vi "config_file_load_create.vi"(0 "configuration file path":path, 1 "reference cluster in":T1, 3 "error in":errorcluster) -> (8 "reference cluster out":T1, 10 "error out":errorcluster)   [LabVIEW 2016]
uses:
  Type Definitions/reference_cluster.ctl
  Type Definitions/vars_settings.ctl
  Type Definitions/stim_type.ctl
  Type Definitions/vars_runtime.ctl
  Type Definitions/data.ctl
  Type Definitions/notifier_elements_GUI.ctl
  Type Definitions/notifier_elements_DAQ.ctl
  Type Definitions/notifier_elements_write.ctl
  Type Definitions/control_references.ctl
  <vilib>/Utility/config.llb/NI_LVConfig.lvlib
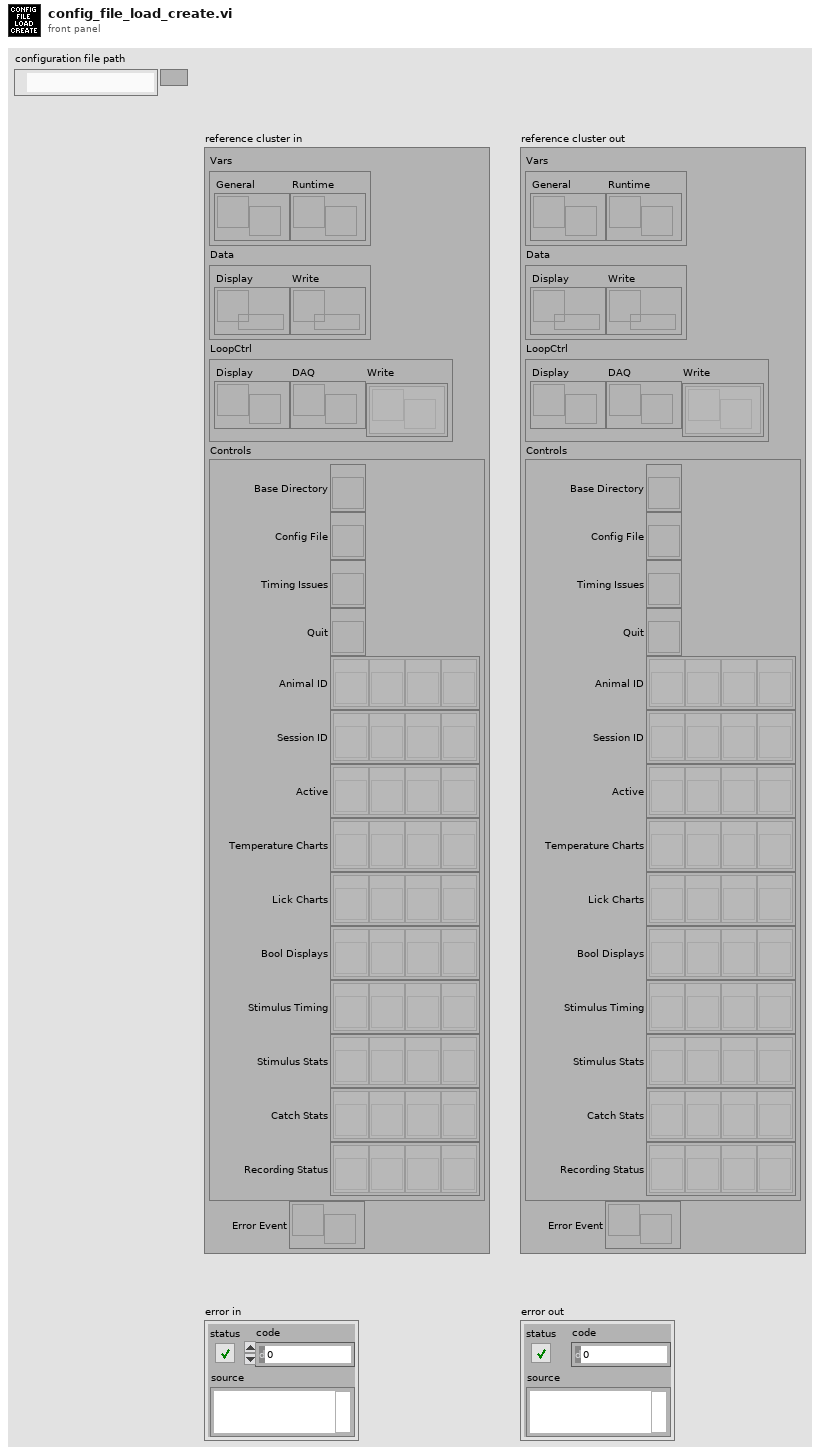
[diagram p1: front panel]
types:
  T1 = typedef "reference_cluster.ctl" = cluster{"Vars":cluster{"General":refnum<notifier>, "Runtime":refnum<notifier>}, "Data":cluster{"Display":refnum<queue>, "Write":refnum<queue>}, "LoopCtrl":cluster{"Display":refnum<notifier>, "DAQ":refnum<notifier>, "Write":refnum<notifier>[]}, "Controls":T2, "Error Event":refnum<user-event>}
  T2 = typedef "control_references.ctl" = cluster{"Base Directory":refnum<vi>, "Config File":refnum<vi>, "Timing Issues":refnum<vi>, "Quit":refnum<vi>, "Animal ID":refnum<vi>[], "Session ID":refnum<vi>[], "Active":refnum<vi>[], "Temperature Charts":refnum<vi>[], "Lick Charts":refnum<vi>[], "Bool Displays":refnum<vi>[], "Stimulus Timing":refnum<vi>[], "Stimulus Stats":refnum<vi>[], "Catch Stats":refnum<vi>[], "Recording Status":refnum<vi>[]}
  T3 = typedef "vars_settings.ctl" = cluster{"base directory":path, "data directory":path, "active":bool, "running":bool, "pairing":bool, "clean tubes":bool, "animal ID":u16, "session ID":u16, "base temp":dbl, "d wait min":u16, "d wait max":u16, "d timeout":u16, "d reward":u16, "idx stim":u16, "timeout win":u16, "lick win":i32[], "stim type":T4[], "stim amps":dbl[], "d stim":u16[], "d ramp":u16[], "f vibration":u16[], "f squarewave":u8[], "stim shape":dbl[][], "catch":u8[]}
  T4 = typedef "stim_type.ctl" = enum16{"pulse", "vibration", "square", "sine"}
  T5 = typedef "NI_LVConfig.lvlib/Config Data RefNum.ctl" = refnum<k1>
  T6 = cluster{"animal ID":u16, "active":bool, "base temp":dbl, "d wait min":u16, "d wait max":u16, "d stim":u16[], "d ramp":u16[], "d timeout":u16, "d reward":u16, "timeout win":u16, "lick win":i32[], "stim amps":dbl[], "catch":u8[], "stim type":T4[], "f vibration":u16[], "f squarewave":u8[]}
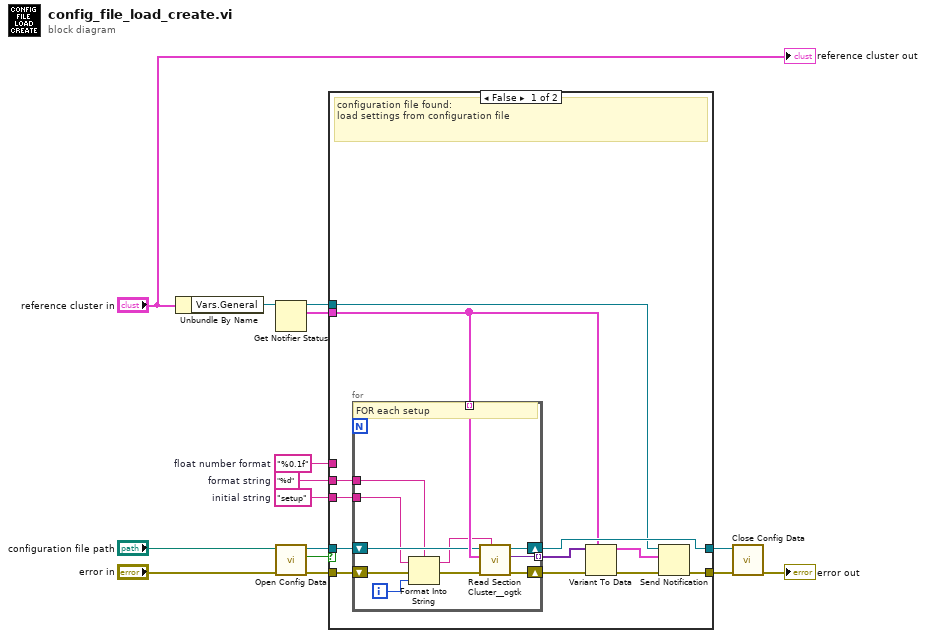
[diagram p0: block diagram]
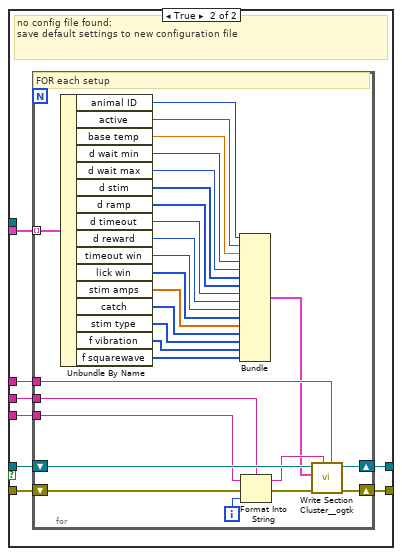
[diagram p2: hidden frame]
diagram:
  w14 = "%0.1f"  # float number format
  w13 = "%d"  # format string
  w12 = "setup"  # initial string
  n1 = Unbundle By Name("reference cluster in") -> ("Vars.General"=w9:refnum<notifier>)
  n2 = Get Notifier Status(notifier=w9) -> (notifier out=w11:refnum<notifier>, current notification=w10:T3[])  [unwired: 1 in, 3 out]
  n3 = call <vilib>:"Open Config Data.vi"("error in (no error)"="error in", "configuration file path"="configuration file path") -> ("error out"=w4:errorcluster, "file created?"=w3:bool, "refnum"=w2:T5)  [unwired: 7 in]
  n4 = case shown="False" w3 {
    tunnel: w4 -> [w26 w46]
    tunnel: [w18 w40] -> w7
    tunnel: w2 -> [w25 w45]
    tunnel: [w27 w41] -> w8
    tunnel: w10 -> [w20 w42]
    tunnel: w11 -> [w16 _]
    tunnel: w12 -> [w24 w44]
    tunnel: w13 -> [w23 w43]
    tunnel: w14 -> [_ w39]
    frame False {
      # "configuration file found:\nload settings from configuration file"
      n5 = for {
        tunnel: [w28] -> w22 mode=indexing
        shift-right: [w35] -> w21
        shift-left: w26 -> [w31]
        shift-right: [w34] -> w27
        shift-left: w25 -> [w36]
        tunnel: w24 -> [w32]
        tunnel: w23 -> [w30]
        tunnel: w20 -> [w38] mode=indexing
        i -> [w33]
        # "FOR each setup"
        n6 = Format Into String(format string=w30, initial string=w32, error in=w31, w33) -> (resulting string=w29:string, error out=w37:errorcluster)
        n7 = call <userlib>:"Read Section Cluster__ogtk.vi"("section (optional)"=w29, "error in (no error)"=w37, "Section Formatted Cluster Type"=w38, "refnum"=w36) -> ("error out"=w35:errorcluster, "Section Formatted Cluster"=w28:variant, "dup refnum"=w34:T5)  [unwired: 3 in, 2 out]
      }
      n8 = Variant To Data(error in=w21, type=w20, Variant=w22) -> (data=w17:T3[], error out=w19:errorcluster)
      n9 = Send Notification(notification=w17, notifier=w16, error in (no error)=w19) -> (error out=w18:errorcluster)  [unwired: 1 out]
    }
    frame True {
      # "no config file found:\nsave default settings to new configuration file"
      n10 = for {
        tunnel: w42 -> [w64] mode=indexing
        shift-right: [w72] -> w40
        shift-left: w46 -> [w68]
        shift-right: [w71] -> w41
        shift-left: w45 -> [w73]
        tunnel: w44 -> [w69]
        tunnel: w43 -> [w67]
        tunnel: w39 -> [w65]
        i -> [w70]
        # "FOR each setup"
        n11 = Unbundle By Name(w64) -> ("animal ID"=w51:u16, "active"=w61:bool, "base temp"=w63:dbl, "d wait min"=w60:u16, "d wait max"=w59:u16, "d stim"=w58:u16[], "d ramp"=w52:u16[], "d timeout"=w57:u16, "d reward"=w53:u16, "timeout win"=w56:u16, "lick win"=w55:i32[], "stim amps"=w54:dbl[], "catch"=w50:u8[], "stim type"=w48:T4[], "f vibration"=w49:u16[], "f squarewave"=w47:u8[])
        n12 = Bundle("animal ID"=w51, "active"=w61, "base temp"=w63, "d wait min"=w60, "d wait max"=w59, "d stim"=w58, "d ramp"=w52, "d timeout"=w57, "d reward"=w53, "timeout win"=w56, "lick win"=w55, "stim amps"=w54, "catch"=w50, "stim type"=w48, "f vibration"=w49, "f squarewave"=w47) -> (w62:T6)  [unwired: 1 in]
        n13 = Format Into String(format string=w67, initial string=w69, error in=w68, w70) -> (resulting string=w66:string, error out=w74:errorcluster)
        n14 = call <userlib>:"Write Section Cluster__ogtk.vi"("float number format (optional)"=w65, "section (optional)"=w66, "error in (no error)"=w74, "Section Formatted Cluster"=w62, "refnum"=w73) -> ("error out"=w72:errorcluster, "dup refnum"=w71:T5)  [unwired: 5 in]
      }
    }
  }
  n15 = call <vilib>:"Close Config Data.vi"("error in (no error)"=w7, "refnum"=w8) -> ("error out"=→"error out":errorcluster)  [unwired: 8 in, 1 out]
  "reference cluster out" <- "reference cluster in"
